vi "GetIntersectionOfLines.vi"(2 "Line1Idx":i32, 3 "Line0Idx":i32, 4 "InterceptArray":dbl[][](array[numeric]), 5 "SlopeArray":dbl[][](array[numeric])) -> (0 "Y":dbl, 1 "X":dbl)   [LabVIEW 2019]
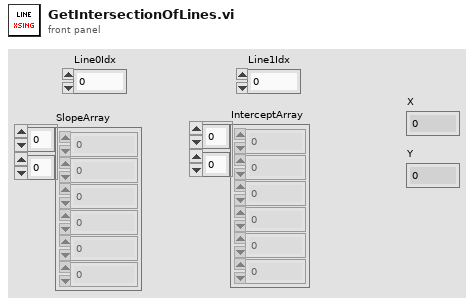
[diagram p1: front panel]
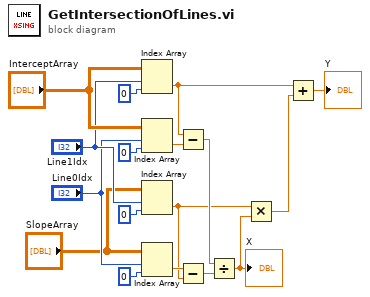
[diagram p0: block diagram]
diagram:
  n1 = Index Array(array="InterceptArray", index (row)="Line1Idx", index (col)=0 ("disabled index (col)")) -> (element=w10:dbl)
  n2 = Index Array(array="InterceptArray", index (row)="Line0Idx", index (col)=0 ("disabled index (col)")) -> (element=w16:dbl)
  n3 = Index Array(array="SlopeArray", index (row)="Line1Idx", index (col)=0 ("disabled index (col)")) -> (element=w12:dbl)
  n4 = Index Array(array="SlopeArray", index (row)="Line0Idx", index (col)=0 ("disabled index (col)")) -> (element=w17:dbl)
  n5 = Subtract(x=w10, y=w16) -> (x-y=w13:dbl)
  n6 = Subtract(x=w17, y=w12) -> (x-y=w14:dbl)
  n7 = Divide(x=w13, y=w14) -> (x/y=w11:dbl)
  "X" <- w11
  n8 = Multiply(x=w12, y=w11) -> (x*y=w9:dbl)
  n9 = Add(x=w10, y=w9) -> (x+y=→"Y":dbl)
